vi "Email_List.vi"(1 "Name Ring Out":u16(ring) items=["Jeremy", "Pete"], 8 "Open File":bool, 10 "List Location":path, 11 "Text Editor Location":path) -> (0 "String":string, 9 "Name Ring In":u16(ring) items=["Jeremy", "Pete"])   [LabVIEW 2011]
uses:
  <vilib>/Utility/file.llb/Write To Spreadsheet File (string).vi
  <vilib>/Utility/file.llb/Read From Spreadsheet File (string).vi
panel:
  in  "command line 1":string="notepad LabVIEW.ini"
  in  "Boolean":bool
  out "Array":string[][](array[string])
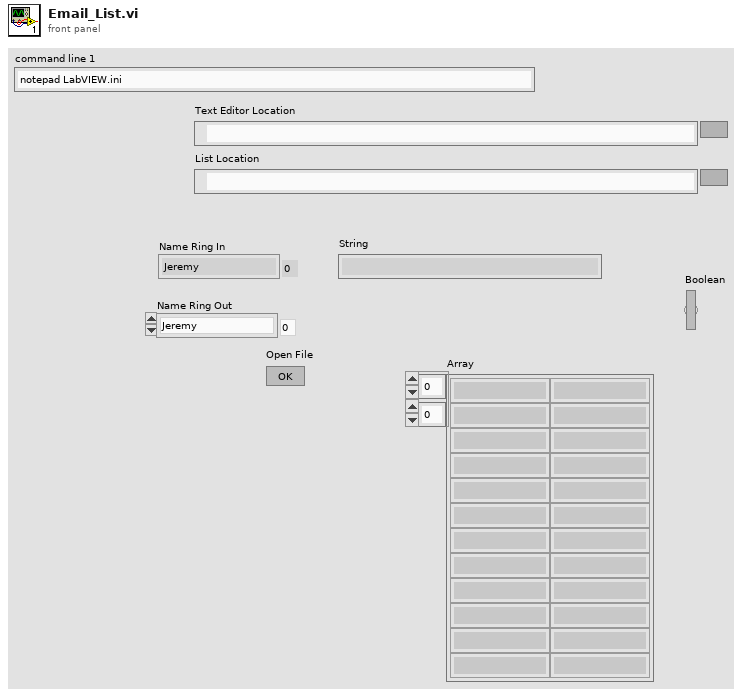
[diagram p1: front panel]
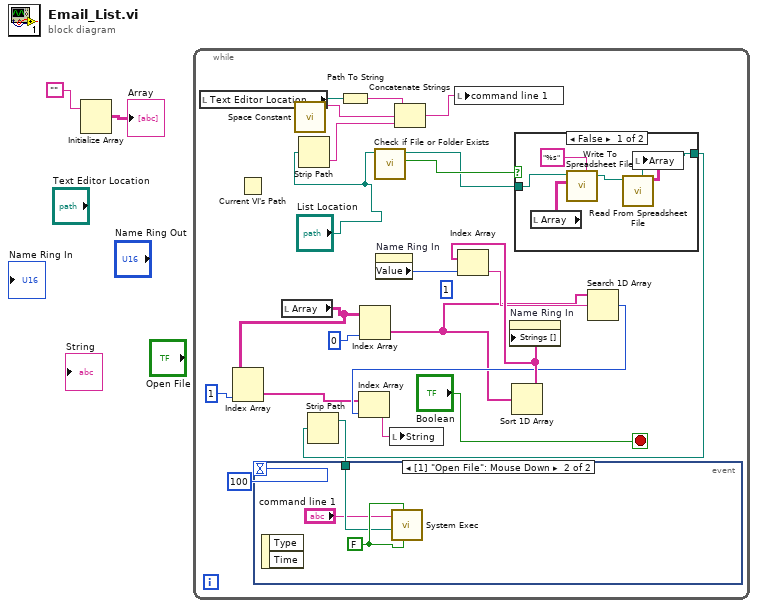
[diagram p0: block diagram]
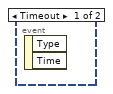
[diagram p2: hidden frame]
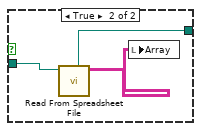
[diagram p3: hidden frame]
diagram:
  n1 = Initialize Array("") -> (→"Array":string[][])  [unwired: 2 in]
  n2 = while {
    stop <- "Boolean" stop-if-true
    (unwired) 1
    n3 = local read "Text Editor Location"() -> (w9:path)
    n4 = Current VI's Path() -> ()  [unwired: 1 out]
    n5 = local read "Array"() -> (w14:string[][])
    n6 = Index Array(array=w14, index (col)=1) -> (element=w12:string[])  [unwired: 1 in]
    n7 = call <vilib>:"Space Constant.vi"() -> ("String"=w5:string)
    n8 = Strip Path(path="List Location") -> (name=w6:string)  [unwired: 1 out]
    n9 = Path To String(path=w9) -> (string=w8:string)
    n10 = Index Array(array=w14, index (col)=0) -> (element=w15:string[])  [unwired: 1 in]
    n11 = call <vilib>:"Check if File or Folder Exists.vi"("path"="List Location") -> ("file or folder exists?"=w24:bool, "dup path"=w23:path)  [unwired: 8 in, 1 out]
    n12 = property on="Name Ring In" class="Ring (strict)"() -> ("Value"=w20:u16)  [unwired: 2 in, 2 out]
    n13 = Concatenate Strings(w8, w5, w6) -> (w4:string)
    n14 = local write "command line 1"(w4) -> ()
    n15 = Sort 1D Array(array=w15) -> (sorted array=w19:string[])
    n16 = Index Array(array=w19, index=w20) -> (element=w18:string)
    n17 = property on="Name Ring In" class="Ring (strict)"("Strings []"=w19) -> ()  [unwired: 2 in, 2 out]
    n18 = case shown="False" w24 {
      tunnel: w23 -> [w33 w36]
      tunnel: [w28 w34] -> w3
      frame False {
        n19 = local read "Array"() -> (w30:string[][])
        n20 = call-poly <vilib>:"Write To Spreadsheet File.vi"("format (%s)"="%s", "2D data"=w30, "file path (dialog if empty)"=w33) -> ("new file path (Not A Path if cancelled)"=w32:path)  [unwired: 5 in]
        n21 = call-poly <vilib>:"Read From Spreadsheet File.vi"("file path (dialog if empty)"=w32) -> ("all rows"=w29:string[][], "new file path (Not A Path if cancelled)"=w28:path)  [unwired: 6 in, 3 out]
        n22 = local write "Array"(w29) -> ()
      }
      frame True {
        n23 = call-poly <vilib>:"Read From Spreadsheet File.vi"("file path (dialog if empty)"=w36) -> ("all rows"=w35:string[][], "new file path (Not A Path if cancelled)"=w34:path)  [unwired: 6 in, 3 out]
        n24 = local write "Array"(w35) -> ()
      }
    }
    n25 = Strip Path(path=w3) -> (stripped path=w10:path)  [unwired: 1 out]
    n26 = event shown="[1] \"Open File\": Mouse Down" {
      selector: _ -> [_ _]
      dyn-events: _ -> [_ _]
      timeout: 100 -> [_ _]
      tunnel: w10 -> [_ w26]
      event Timeout {
        n27 = event-data() -> ()  [unwired: 1 in, 2 out]
      }
      event "Open File": Mouse Down {
        w27 = FALSE
        n28 = event-data() -> ()  [unwired: 1 in, 2 out]
        n29 = call <vilib>:"System Exec.vi"("run minimized? (F)"=w27, "wait until completion? (T)"=w27, "working directory"=w26, "command line"="command line 1") -> ()  [unwired: 2 in, 6 out]
      }
    }
    n30 = Search 1D Array(1D array=w15, element=w18) -> (index of element=w16:i32)  [unwired: 1 in]
    n31 = Index Array(array=w12, index=w16) -> (element=w17:string)
    n32 = local write "String"(w17) -> ()
  }
